vi "Eurotherm - VISA Serial - Clear Buffer.vi"(0 "VISA resource name":refnum<visa-resource-name>, 11 "error in (no error)":errorcluster) -> (4 "dup VISA resource name":refnum<visa-resource-name>, 15 "error out":errorcluster)   [LabVIEW 2011]
panel:
  out "return count":u32
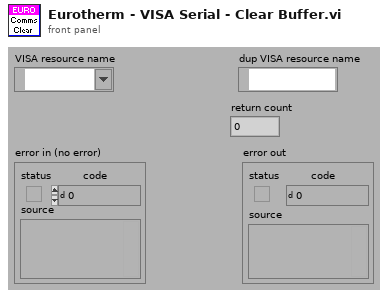
[diagram p1: front panel]
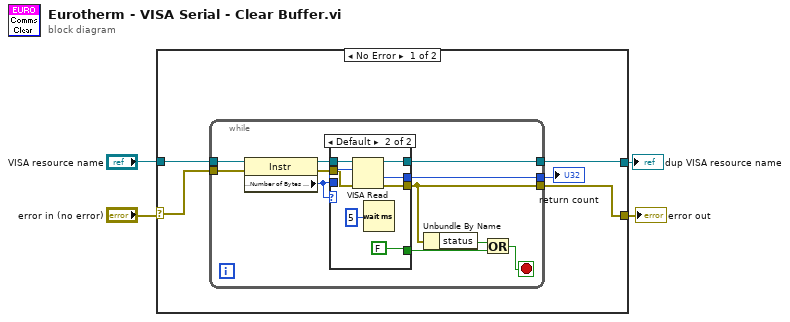
[diagram p0: block diagram]
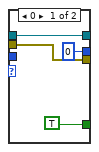
[diagram p2: hidden frame]
diagram:
  n1 = case shown="No Error" "error in (no error)" {
    selector: "error in (no error)" -> [w8 w34]
    tunnel: [w7 w34] -> w3
    tunnel: "VISA resource name" -> [w9 w33]
    tunnel: [w6 w33] -> w1
    frame No Error {
      n2 = while {
        tunnel: w9 -> [w18]
        tunnel: w8 -> [w17]
        tunnel: [w13] -> w7
        tunnel: [w15] -> w6
        tunnel: [w14] -> w5
        stop <- w10 stop-if-true
        n3 = property class="Instr"(reference=w18, error in=w17) -> (reference out=w20:refnum<visa-resource-name>, error out=w19:errorcluster, "Serial Settings:Number of Bytes at Serial Port"=w16:u32)
        n4 = case shown="Default" w16 {
          tunnel: w20 -> [w23 w32]
          tunnel: w16 -> [_ w31]
          tunnel: w19 -> [w24 w30]
          tunnel: [w24 w29] -> w13
          tunnel: [w23 w28] -> w15
          tunnel: [u32 0 ("return count") w27] -> w14
          tunnel: [TRUE FALSE] -> w11
          frame 0 {
          }
          frame Default {
            n5 = VISA Read(VISA resource name=w32, byte count=w31, error in (no error)=w30) -> (VISA resource name out=w28:refnum<visa-resource-name>, return count=w27:u32, error out=w29:errorcluster)  [unwired: 1 out]
            n6 = Wait (ms)(milliseconds to wait=u32 5) -> ()  [unwired: 1 out]
          }
        }
        n7 = Unbundle By Name(w13) -> ("status"=w12:bool)
        n8 = Or(x=w12, y=w11) -> (x .or. y?=w10:bool)
      }
      "return count" <- w5
    }
    frame Error {
    }
  }
  "error out" <- w3
  "dup VISA resource name" <- w1
